vi "Load JSON Teams in Match Number.vi"(9 "Match":i32, 10 "All Files in Dir":path[](array[path]), 11 "ListBox in":refnum<vi>) -> ()   [LabVIEW 2015]
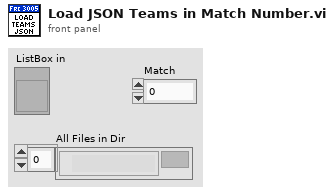
[diagram p1: front panel]
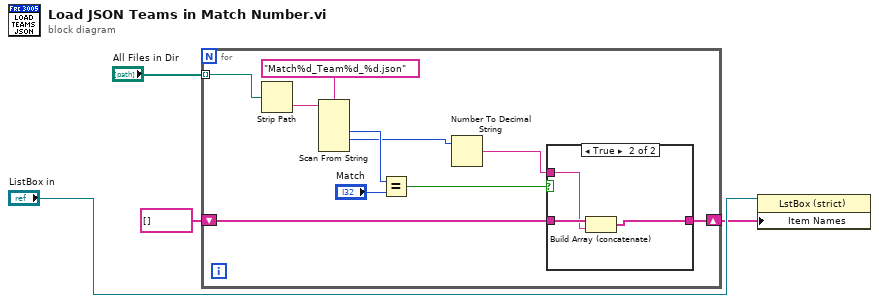
[diagram p0: block diagram]
diagram:
  n1 = for {
    tunnel: "All Files in Dir" -> [w14] mode=indexing
    shift-right: [w11] -> w2
    shift-left: string[] [] -> [w7]
    n2 = Strip Path(path=w14) -> (name=w13:string)  [unwired: 1 out]
    n3 = Scan From String(format string="Match%d_Team%d_%d.json", input string=w13) -> (output 1=w9:i32, output 2=w6:i32)  [unwired: 6 in, 3 out]
    n4 = Equal?(x=w9, y="Match") -> (x = y?=w8:bool)
    n5 = Number To Decimal String(number=w6) -> (decimal integer string=w5:string)  [unwired: 1 in]
    n6 = case shown="True" w8 {
      tunnel: [w15 w18] -> w11
      tunnel: w7 -> [w15 w17]
      tunnel: w5 -> [_ w16]
      frame False {
      }
      frame True {
        n7 = Build Array (concatenate)(w17, w16) -> (w18:string[])
      }
    }
  }
  n8 = property class="LstBox (strict)"(reference="ListBox in", "Item Names"=w2) -> ()  [unwired: 1 in, 2 out]
